vi "SignProviderINIFiles.vi"() -> ()   [LabVIEW 2012]
panel:
  out "Error Out":errorcluster
  # "This VI will sign one or all project provider  INI files in a directory.  It will create INI files in the same directory with or without \"_signed\" appended to the file name."
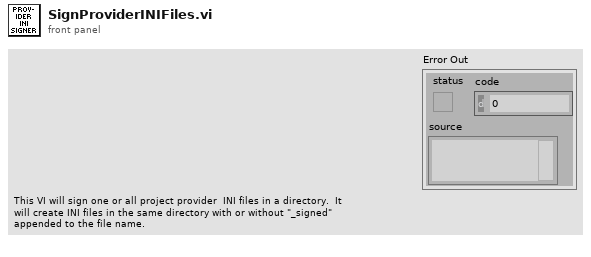
[diagram p1: front panel]
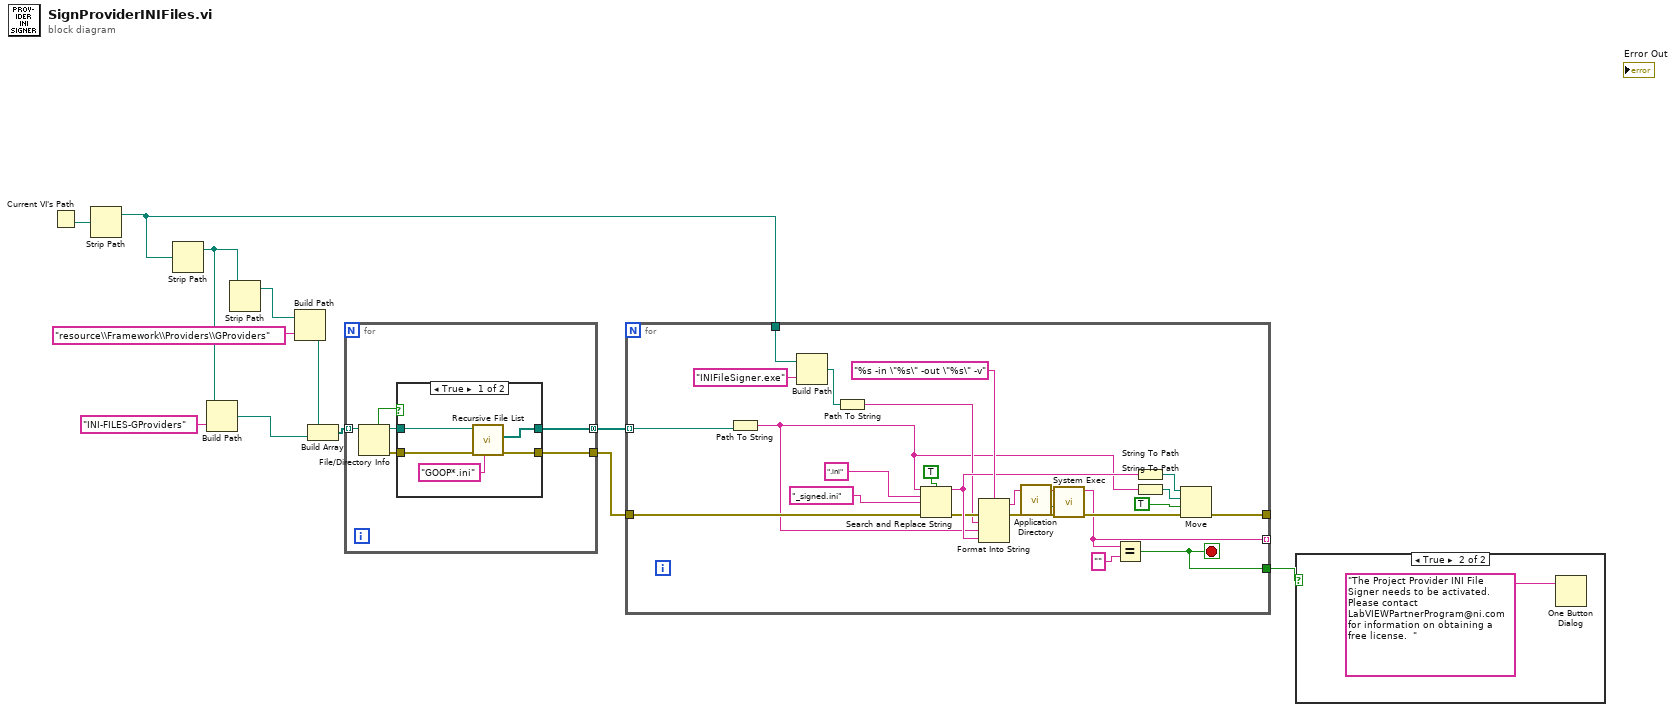
[diagram p0: block diagram]
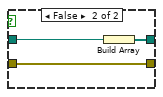
[diagram p2: hidden frame]
diagram:
  n1 = Current VI's Path() -> (path=w2:path)
  n2 = Strip Path(path=w2) -> (stripped path=w1:path)  [unwired: 1 out]
  n3 = Strip Path(path=w1) -> (stripped path=w7:path)  [unwired: 1 out]
  n4 = Build Path(base path=w7, name or relative path="INI-FILES-GProviders") -> (appended path=w4:path)
  n5 = Strip Path(path=w7) -> (stripped path=w8:path)  [unwired: 1 out]
  n6 = Build Path(base path=w8, name or relative path="resource\\Framework\\Providers\\GProviders") -> (appended path=w9:path)
  n7 = Build Array(w9, w4) -> (w5:path[])
  n8 = for {
    tunnel: [w15] -> w11
    tunnel: w5 -> [w14] mode=indexing
    tunnel: [w13] -> w3 mode=concatenating
    n9 = File/Directory Info(path=w14) -> (path out=w16:path, directory=w17:bool, error out=w18:errorcluster)  [unwired: 1 in, 4 out]
    n10 = case shown="True" w17 {
      tunnel: w16 -> [w21 w24]
      tunnel: [w22 w26] -> w13
      tunnel: w18 -> [w20 w25]
      tunnel: [w19 w25] -> w15
      frame True {
        n11 = call <vilib>:"Recursive File List.vi"("pattern"="GOOP*.ini", "error in (no error)"=w20, "Folder Path"=w21) -> ("error out"=w19:errorcluster, "All Files in Dir"=w22:path[])  [unwired: 4 in, 3 out]
      }
      frame False {
        n12 = Build Array(w24) -> (w26:path[])
      }
    }
  }
  n13 = for {
    tunnel: [w36] -> _ mode=indexing
    tunnel: w11 -> [w41]
    tunnel: [w40] -> _
    tunnel: [w32] -> w12
    tunnel: w1 -> [w28]
    tunnel: w3 -> [w27] mode=indexing
    stop <- w32 stop-if-true
    n14 = Path To String(path=w27) -> (string=w34:string)
    n15 = Build Path(base path=w28, name or relative path="INIFileSigner.exe") -> (appended path=w39:path)
    n16 = Path To String(path=w39) -> (string=w35:string)
    n17 = Search and Replace String(case sensitive?=TRUE ("ignore case? (F)"), input string=w34, search string=".ini" ("regular expression"), replace string="_signed.ini" ("string"), error in=w41) -> (result string=w45:string, error out=w43:errorcluster)  [unwired: 3 in, 2 out]
    n18 = Format Into String(format string="%s -in \"%s\" -out \"%s\" -v", error in=w43, w35, w34, w45) -> (resulting string=w49:string, error out=w42:errorcluster)  [unwired: 1 in]
    n19 = call <vilib>:"Application Directory.vi"() -> ("Application Directory"=w33:path)
    n20 = call <vilib>:"System Exec.vi"("error in (no error)"=w42, "working directory"=w33, "command line"=w49) -> ("error out"=w44:errorcluster, "standard output"=w36:string)  [unwired: 5 in, 2 out]
    n21 = Equal?(x=w36, y="") -> (x = y?=w32:bool)
    n22 = String To Path(string=w45) -> (path=w31:path)
    n23 = String To Path(string=w34) -> (path=w30:path)
    n24 = Move(source path=w31, error in=w44, 9:TRUE ("overwrite (F)"), 10:w30) -> (error out=w40:errorcluster)  [unwired: 1 in, 2 out]
  }
  n25 = case shown="True" w12 {
    frame False {
    }
    frame True {
      n26 = One Button Dialog(message="The Project Provider INI File Signer needs to be activated.  Please contact LabVIEWPartnerProgram@ni.com for information on obtaining a free license.  ") -> ()  [unwired: 1 in, 1 out]
    }
  }
